vi "Main.vi"() -> ()   [LabVIEW 2023]
uses:
  <vilib>/MakerHub/LINX/Public/Utilities/Open Serial.vi
  <vilib>/MakerHub/LINX/Public/Sensors/Motion/Servo/Servo Open One Channel.vi
  <vilib>/MakerHub/LINX/Public/Sensors/Motion/Servo/Servo Set Pulse Width One Channel.vi
  <vilib>/MakerHub/LINX/Public/Sensors/Motion/Servo/Servo Close One Channel.vi
  <vilib>/MakerHub/LINX/LMH-LINX.lvlib
  <vilib>/MakerHub/LINX/Public/Sensors/Motion/Servo/Servo.lvlib
panel:
  out "Device Name":string
  in  "Stop Button":bool
  out "Pulse Width uS":dbl
  out "Angle":dbl
  in  "Period":u32
  in  "Serial Port":refnum<visa-resource-name>="N/A"
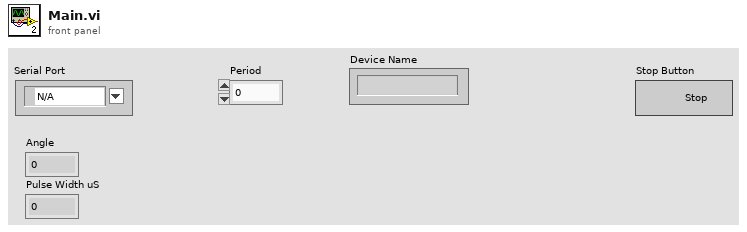
[diagram p1: front panel]
types:
  T1 = typedef "LMH-LINX.lvlib/LINX Ref.ctl" = cluster{"IO":T2, "Interface":T3, "LINX Device Config":T4}
  T2 = typedef "LMH-LINX.lvlib/Platform.ctl" = enum16{"Remote", "Local"}
  T3 = typedef "LMH-LINX.lvlib/Interface.ctl" = enum16{"Serial", "TCP"}
  T4 = typedef "LMH-LINX.lvlib/Device.lvlib/LINX Device Config.ctl" = cluster{"Interface":T3, "COM Port":refnum<visa-resource-name>, "TCP Configuration":T5, "Device Family":u8, "Device ID":u8, "Device Name":string, "TCP Ref":refnum<k5>, "Channels":T6}
  T5 = typedef "LMH-LINX.lvlib/Device.lvlib/TCP Config.ctl" = cluster{"IP Address":string, "Port":u16}
  T6 = typedef "LMH-LINX.lvlib/Channels.ctl" = cluster{"DI":u8[], "DO":u8[], "AI":u8[], "AO":u8[], "PWM":u8[], "QE":u8[], "UART":u8[], "I2C 2":u8[], "SPI":u8[], "CAN":u8[], "Servo":u8[], "AI Ref (V)":dbl, "AI Resolution (Bits)":u8, "AO Ref (V)":dbl, "AO Resolution (Bits)":u8}
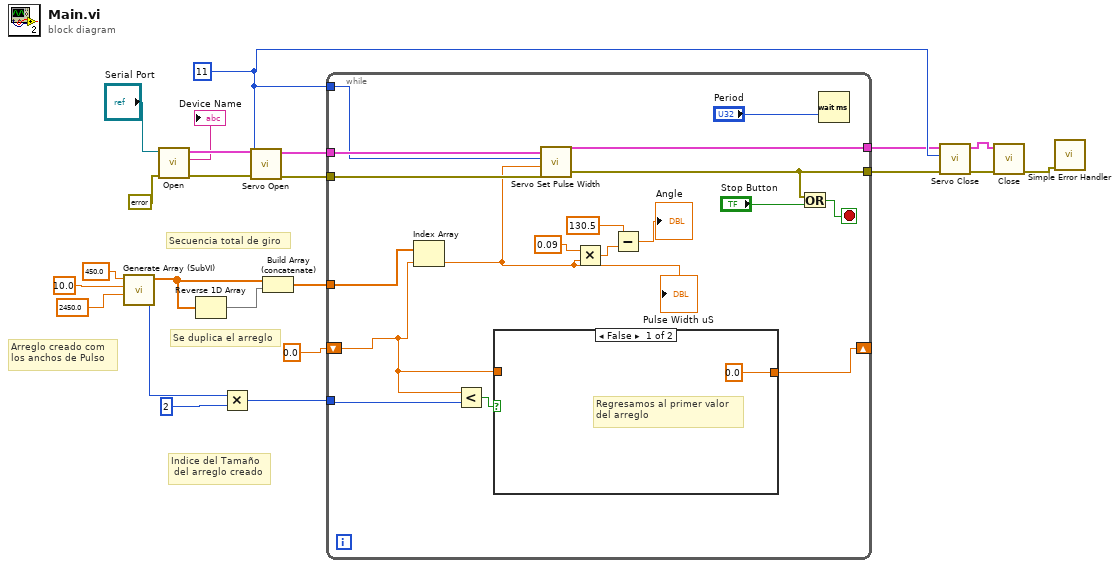
[diagram p0: block diagram]
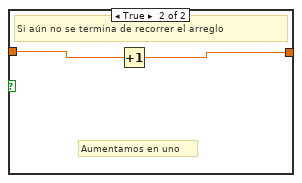
[diagram p2: hidden frame]
diagram:
  w17 = u8 11 ("Servo Channel")
  # "Arreglo creado com\nlos anchos de Pulso"
  # "Indice del Tamaño\n del arreglo creado"
  # "Se duplica el arreglo"
  # "Secuencia total de giro"
  n1 = call "Generate Array (SubVI).vi"("Final"=2450.0, "Step"=10.0, "Initial"=450.0) -> ("Array size"=w5:i32, "Array out"=w8:dbl[])  [unwired: 6 in, 1 out]
  n2 = call-poly <vilib>:"Open.vi"("Error In"=errorcluster {"status"=FALSE, "code"=0, "source"=""}, "Serial Port"="Serial Port") -> ("Error Out"=w22:errorcluster, "Device Name"=→"Device Name":string, "LINX Resource"=w23:T1)  [unwired: 7 in]
  n3 = Reverse 1D Array(array=w8) -> (reversed array=w7:dbl[])
  n4 = Multiply(x=w5, y=2) -> (x*y=w3:i32)
  n5 = call-poly <vilib>:"Servo Open.vi"("Error In"=w22, "Servo Channel"=w17, "LINX Resource"=w23) -> ("Error Out"=w20:errorcluster, "LINX Resource"=w21:T1)  [unwired: 7 in]
  n6 = Build Array (concatenate)(w8, w7) -> (w6:dbl[])
  n7 = while {
    tunnel: w21 -> [w41]
    tunnel: w20 -> [w40]
    tunnel: w17 -> [w39]
    tunnel: [w38] -> w16
    tunnel: [w26] -> w15
    shift-right: [w27] -> _
    shift-left: 0.0 -> [w28]
    tunnel: w6 -> [w33]
    tunnel: w3 -> [w30]
    stop <- w24 stop-if-true
    n8 = Index Array(array=w33, index=w28) -> (element=w32:dbl)
    "Pulse Width uS" <- w32
    n9 = Less?(x=w28, y=w30) -> (x < y?=w29:bool)
    n10 = case shown="False" w29 {
      tunnel: w28 -> [_ w44]
      tunnel: [0.0 w43] -> w27
      frame False {
        # "Regresamos al primer valor \ndel arreglo"
      }
      frame True {
        # "Aumentamos en uno"
        # "Si aún no se termina de recorrer el arreglo"
        n11 = Increment(x=w44) -> (x+1=w43:dbl)
      }
    }
    n12 = call-poly <vilib>:"Servo Set Pulse Width.vi"("Error In"=w40, "Pulse Width (uS)"=w32, "Servo Channel"=w39, "LINX Resource"=w41) -> ("Error Out"=w26:errorcluster, "LINX Resource"=w38:T1)  [unwired: 6 in]
    n13 = Multiply(x=0.09, y=w32) -> (x*y=w35:dbl)
    n14 = Subtract(x=130.5, y=w35) -> (x-y=→"Angle":dbl)
    n15 = Or(x=w26, y="Stop Button") -> (x .or. y?=w24:bool)
    n16 = Wait (ms)(milliseconds to wait="Period") -> ()  [unwired: 1 out]
  }
  n17 = call-poly <vilib>:"Servo Close.vi"("Error In"=w15, "Servo Channel"=w17, "LINX Resource"=w16) -> ("Error Out"=w13:errorcluster, "LINX Resource"=w14:T1)  [unwired: 7 in]
  n18 = call <vilib>:"Close.vi"("Error In"=w13, "LINX Resource"=w14) -> ("Error Out"=w2:errorcluster)  [unwired: 9 in]
  n19 = call <vilib>:"Simple Error Handler.vi"("error in (no error)"=w2) -> ()  [unwired: 4 in, 5 out]
